vi "`qwr.vi"() -> ()   [LabVIEW 2017]
uses:
  <vilib>/userdefined/High Color/IMAQdx.ctl
  <vilib>/vision/driver/NI_Vision_Acquisition_Software.lvlib
panel:
  out "Image":T1(plugin-control)
  in  "stop":bool
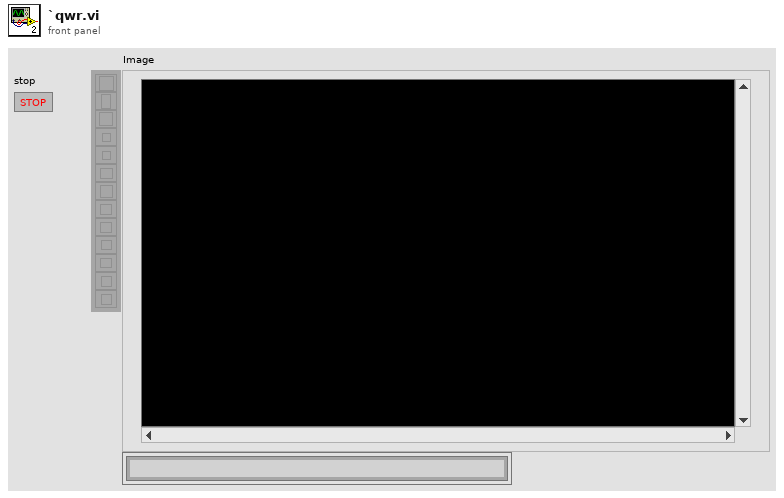
[diagram p1: front panel]
types:
  T1 = typedef "IMAQ Image.ctl" = refnum<image>
  T2 = typedef "IMAQdx.ctl" = refnum<k21>
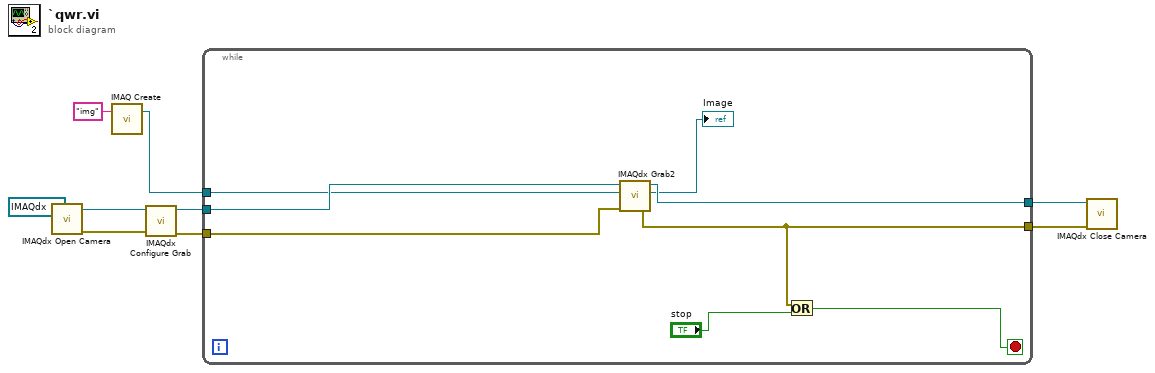
[diagram p0: block diagram]
diagram:
  n1 = call <vilib>:"IMAQdx Open Camera.vi"("Session In"=T2 "cam0") -> ("error out"=w9:errorcluster, "Session Out"=w8:T2)  [unwired: 9 in]
  n2 = call "IMAQ Create"("Image Name"="img") -> ("New Image"=w3:T1)  [unwired: 4 in, 1 out]
  n3 = call <vilib>:"IMAQdx Configure Grab.vi"("error in"=w9, "Session In"=w8) -> ("error out"=w7:errorcluster, "Session Out"=w5:T2)  [unwired: 8 in]
  n4 = while {
    tunnel: w7 -> [w17]
    tunnel: [w14] -> w6
    tunnel: w5 -> [w13]
    tunnel: [w12] -> w4
    tunnel: w3 -> [w11]
    stop <- w16 stop-if-true
    n5 = call <vilib>:"IMAQdx Grab2.vi"("error in"=w17, "Image In"=w11, "Session In"=w13) -> ("error out"=w14:errorcluster, "Image Out"=→"Image":T1, "Session Out"=w12:T2)  [unwired: 5 in, 1 out]
    n6 = Or(x=w14, y="stop") -> (x .or. y?=w16:bool)
  }
  n7 = call <vilib>:"IMAQdx Close Camera.vi"("error in"=w6, "Session In"=w4) -> ()  [unwired: 9 in, 1 out]
